vi "Convert Point 2D (SGL) to Point 2D (I32).vi"(11 "Point 2D (Float)":T2) -> (3 "Point 2D (I32)":T1)   [LabVIEW 2020, in "3D.lvlib"]
uses:
  3D.lvlib
  Point 2D.ctl
  Raster/Point 2D.ctl
  Raster/Raster.lvlib
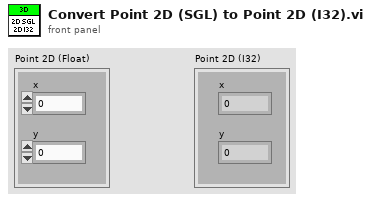
[diagram p1: front panel]
types:
  T1 = typedef "Raster.lvlib/Point 2D.ctl" = cluster{"x":i32, "y":i32}
  T2 = typedef "3D.lvlib/Point 2D.ctl" = cluster{"x":sgl, "y":sgl}
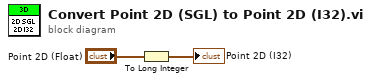
[diagram p0: block diagram]
diagram:
  n1 = To Long Integer(number="Point 2D (Float)") -> (32bit integer=→"Point 2D (I32)":cluster{"x":i32, "y":i32})
